vi "evaluate_waveforms.vi"(8 "error in (no error)":errorcluster, 10 "ExperimentVariables (in)":refnum<class "ExperimentVariables.lvclass">, 11 "HSDIO in":refnum<class "HSDIO.lvclass">) -> (0 "error out":errorcluster, 1 "HSDIO Status":T1, 2 "ExperimentVariables":refnum<class "ExperimentVariables.lvclass">, 3 "HSDIO out":refnum<class "HSDIO.lvclass">)   [LabVIEW 2012, in "HSDIO.lvclass"]
uses:
  HSDIO.lvclass
  ExperimentVariables/ExperimentVariables.lvclass
  HSDIO.lvclass/HSDIO.ctl
  <instrlib>/niHSDIO/niHSDIO.llb/niHSDIO Write Named Waveform (1D U32).vi
  <vilib>/regexp/Match Regular Expression.xnode
panel:
  out "Sample Array":u32[](array[numeric])
  out "Sample":u32
  out "waveform names":string[](array[string])
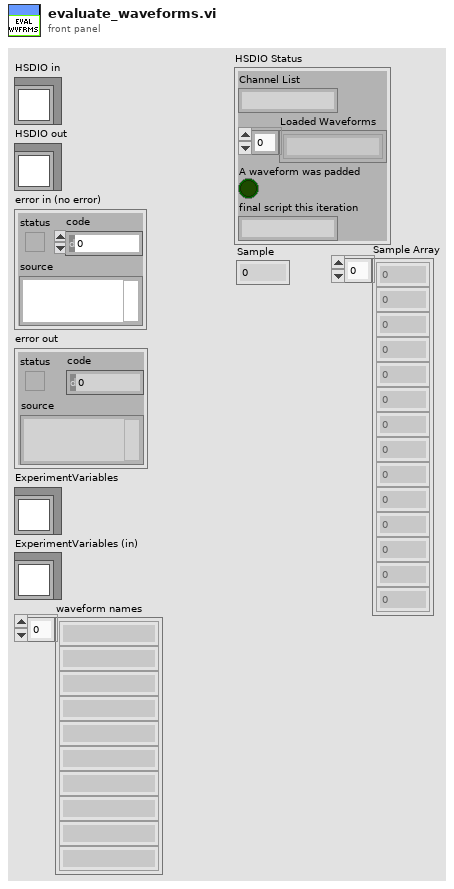
[diagram p1: front panel]
types:
  T1 = cluster{"Channel List":string, "Loaded Waveforms":string[], "A waveform was padded":bool, "final script this iteration":string}
  T2 = typedef "HSDIO.lvclass/HSDIO_settings.ctl" = cluster{"Enable HSDIO Pulses":bool, "Resource Name":refnum<k15>, "Clock Rate":dbl, "units per second":dbl, "Array of Script Triggers":cluster{"trigger id (script trigger 0)":T3, "source (PFI 0)":T4, "Trigger Type":enum32{"Edge", "Level"}, "edge":T5, "level":T6}[], "Channels Control":string[][], "Pulse Generation Script":string, "Directory to look for waveform files:":path, "Start Trigger":cluster{"Wait for start trigger?":bool, "source (PFI 0)":T4, "edge (rising)":T5}, "Hardware alignment quantum (in samples)":u16}
  T3 = typedef "niHSDIO_ctl Trigger Script - trigID Values (Ring).ctl" = string
  T4 = typedef "niHSDIO_ctl Trigger Source Values (Ring).ctl" = string
  T5 = typedef "niHSDIO_ctl Trigger DigEdge - Edge Values (Ring).ctl" = i32
  T6 = typedef "niHSDIO_ctl Trigger DigLvl - Level Values (Ring).ctl" = i32
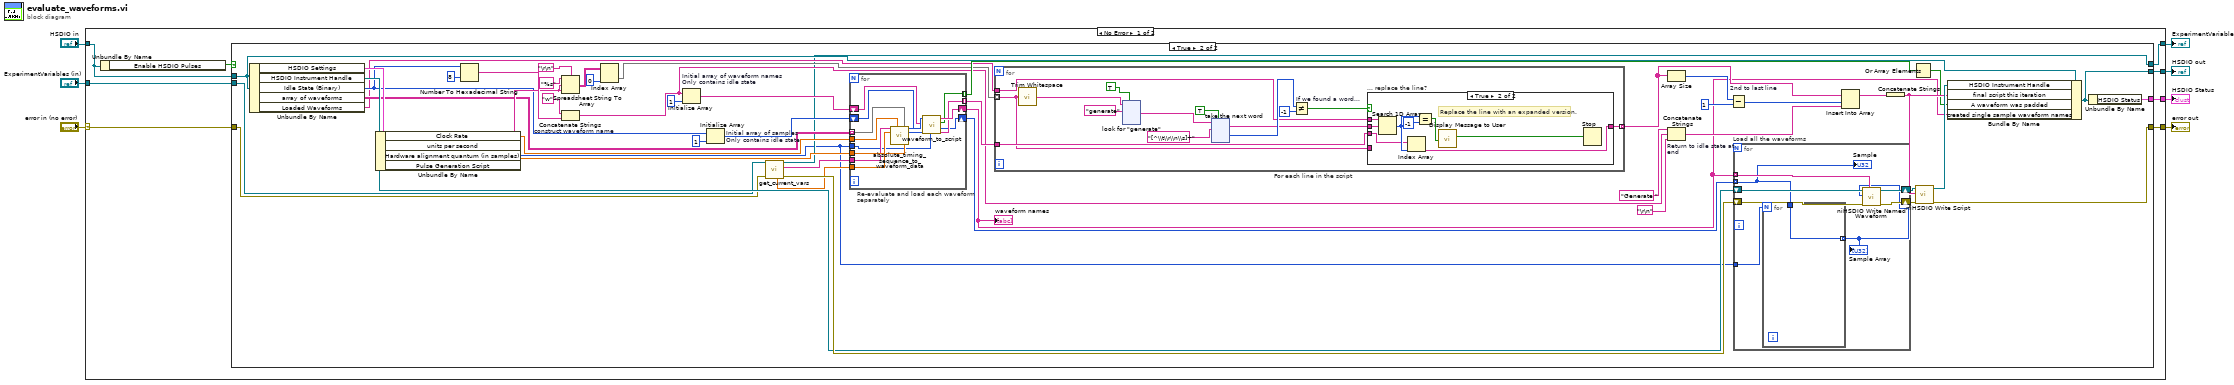
[diagram p0: block diagram]
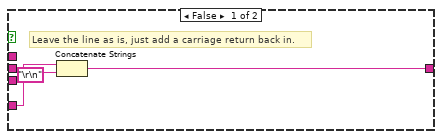
[diagram p3: hidden frame]
diagram:
  n1 = case shown="No Error" "error in (no error)" {
    selector: "error in (no error)" -> [w14 w340]
    tunnel: [w15 w340] -> w6
    tunnel: [w13 w339] -> w4
    tunnel: "HSDIO in" -> [w11 w339]
    tunnel: [w12 _] -> w3
    tunnel: "ExperimentVariables (in)" -> [w9 w338]
    tunnel: [w8 w338] -> w1
    frame No Error {
      n2 = Unbundle By Name(w11) -> ("Enable HSDIO Pulses"=w10:bool)
      n3 = case shown="True" w10 {
        tunnel: [w18 w35] -> w15
        tunnel: w11 -> [w17 w26]
        tunnel: w14 -> [w18 w25]
        tunnel: [w17 w24] -> w13
        tunnel: [_ w23] -> w12
        tunnel: w9 -> [w16 w22]
        tunnel: [w16 w21] -> w8
        frame False {
        }
        frame True {
          n4 = Unbundle By Name(w26) -> ("HSDIO Settings"=w31:T2, "HSDIO Instrument Handle"=w30:refnum<k15>, "Idle State (Binary)"=w29:u32, "array of waveforms"=w28:string[][][], "Loaded Waveforms"=w27:string[])
          n5 = Unbundle By Name(w31) -> ("Clock Rate"=w40:dbl, "units per second"=w37:dbl, "Hardware alignment quantum (in samples)"=w19:u16, "Pulse Generation Script"=w36:string)
          n6 = Number To Hexadecimal String(1:i16 8 ("width (-)"), 2:w29) -> (0:w54:string)
          n7 = Spreadsheet String To Array(delimiter (Tab)="\r\n", format string="%s", spreadsheet string=w36, array type (2D Dbl)=w36) -> (array=w62:string[][])
          n8 = Concatenate Strings "construct waveform name"("w" ("string"), w54) -> (w50:string)
          n9 = Index Array(array=w62, index (col)=0 ("index (row)")) -> (element=w64:string[])  [unwired: 1 in]
          n10 = Initialize Array "Initial array of waveform names\nOnly contains idle state"(w50, 1 ("dimension size")) -> (w52:string[])
          n11 = Initialize Array "Initial array of samples\nOnly contains idle state"(w29, 1 ("dimension size")) -> (w57:u32[])
          n12 = call-dynamic "get_current_vars.vi"("error in (no error)"=w25, "ExperimentVariables in"=w22) -> ("error out"=w41:errorcluster, "variables and parameter names"=w38:string[], "ExperimentVariables out"=w21:refnum<class "ExperimentVariables.lvclass">, "current variable and parameter values"=w39:dbl[])  [unwired: 4 in, 2 out]
          n13 = for "Re-evaluate and load each waveform separately" {
            tunnel: w28 -> [w337] mode=indexing
            tunnel: w39 -> [w336]
            tunnel: w38 -> [w333]
            tunnel: w40 -> [w335]
            tunnel: [w324] -> w67 mode=indexing
            tunnel: w19 -> [w325]
            tunnel: w37 -> [w334]
            tunnel: [w327] -> w63 mode=indexing
            shift-right: [w330] -> w20
            shift-left: w52 -> [w331]
            shift-right: [w326] -> w42
            shift-left: w57 -> [w328]
            n14 = call "absolute_timing_sequence_to_waveform_data.vi"("Variable Names"=w333, "Clock Rate"=w335, "Timing Sequence Control (ms)"=w337, "Current Value Array"=w336, "units/sec (ms=1000)"=w334) -> ("Transitions"=w332:u32[], "Data"=w329:u32[])  [unwired: 6 in, 3 out]
            n15 = call "waveform_to_script.vi"("Hardware alignment quantum (in samples)"=w325, "Data"=w329, "existing waveform samples (in)"=w328, "existing waveform names"=w331, "Transitions (sorted and reduced)"=w332) -> ("script"=w327:string, "waveform samples (out)"=w326:u32[], "Some sample was padded?"=w324:bool, "waveform names"=w330:string[])  [unwired: 3 in]
          }
          "waveform names" <- w20
          n16 = for "For each line in the script" {
            tunnel: w64 -> [w77] mode=indexing
            tunnel: w63 -> [w79]
            tunnel: w27 -> [w81]
            tunnel: [w80] -> w48 mode=indexing
            n17 = call <vilib>:"Trim Whitespace.vi"("string"=w77) -> ("trimmed string"=w89:string)  [unwired: 1 in]
            n18 = xnode "look for \"generate\""("input string"=w89, "regular expression"="generate", "ignore case? (F)"=TRUE) -> ("after match"=w85:string)  [unwired: 3 in, 4 out]
            n19 = xnode "take the next word"("input string"=w85, "regular expression"="[^\\t\\r\\n\\s]+", "ignore case? (F)"=TRUE) -> ("whole match"=w83:string, "offset past match"=w84:i32)  [unwired: 3 in, 3 out]
            n20 = Not Equal? "If we found a word..."(x=w84, y=-1) -> (x != y?=w82:bool)
            n21 = case "... replace the line?" shown="True" w82 {
              tunnel: w83 -> [_ w101]
              tunnel: [w91 w94] -> w80
              tunnel: w77 -> [w93 _]
              tunnel: w79 -> [_ w95]
              tunnel: w81 -> [_ w100]
              frame False {
                # "Leave the line as is, just add a carriage return back in."
                n22 = Concatenate Strings(w93, "\r\n") -> (w91:string)
              }
              frame True {
                # "Replace the line with an expanded version."
                n23 = Search 1D Array(1D array=w100, element=w101) -> (index of element=w96:i32)  [unwired: 1 in]
                n24 = Index Array(array=w95, index=w96) -> (element=w94:string)
                n25 = Equal?(x=w96, y=-1) -> (x = y?=w98:bool)
                n26 = call "Display Message to User"("Enable"=w98) -> ("OK"=w97:bool)  [unwired: 9 in, 1 out]
                n27 = Stop(stop? (T)=w97) -> ()
              }
            }
          }
          n28 = Array Size(array=w48) -> (size(s)=w47:i32)
          n29 = Concatenate Strings "Return to idle state at end"("Generate " ("string"), w50, "\r\n") -> (w44:string)
          n30 = Subtract "2nd to last line"(x=w47, y=1) -> (x-y=w45:i32)
          n31 = for "Load all the waveforms" {
            tunnel: w20 -> [w71] mode=indexing
            shift-right: [w74] -> w59
            shift-left: w30 -> [w75]
            shift-right: [w72] -> w60
            shift-left: w41 -> [w73]
            tunnel: w42 -> [w69] mode=indexing
            tunnel: w19 -> [w70]
            n32 = for {
              N: w70 -> [_]
              tunnel: w69 -> [w76]
              tunnel: [w76] -> w68 mode=indexing
            }
            "Sample Array" <- w68
            n33 = call-poly <instrlib>:"niHSDIO Write Named Waveform.vi"("waveform name (default:\"\")"=w71, "error in (no error)"=w73, "data"=w68, "instrument handle"=w75) -> ("error out"=w72:errorcluster, "instrument handle out"=w74:refnum<k15>)  [unwired: 6 in]
            "Sample" <- w69
          }
          n34 = Insert Into Array(array=w48, index=w45, new element=w44) -> (w43:string[])
          n35 = Concatenate Strings(w43) -> (w33:string)
          n36 = Or Array Elements(Boolean array=w67) -> (logical OR=w32:bool)
          n37 = call <instrlib>:"niHSDIO Write Script.vi"("error in (no error)"=w60, "script"=w33, "instrument handle"=w59) -> ("error out"=w35:errorcluster, "instrument handle out"=w34:refnum<k15>)  [unwired: 7 in]
          n38 = Bundle By Name(cluster=w26, "HSDIO Instrument Handle"=w34, "final script this iteration"=w33, "A waveform was padded"=w32, "created single sample waveform names"=w20) -> (w24:refnum<class "HSDIO.lvclass">)
          n39 = Unbundle By Name(w24) -> ("HSDIO Status"=w23:T1)
        }
      }
    }
    frame Error {
    }
  }
  "error out" <- w6
  "HSDIO out" <- w4
  "HSDIO Status" <- w3
  "ExperimentVariables" <- w1
